vi "Time 1.1-1.2 comparison.vi"() -> ()   [LabVIEW 2013]
panel:
  out "Fib":i32
  out "Time3":dbl
  out "Time2":dbl
  out "f(n)":i32
  out "fib(n)":i32
  out "Time1":dbl
  in  "n":i16
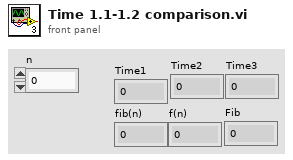
[diagram p1: front panel]
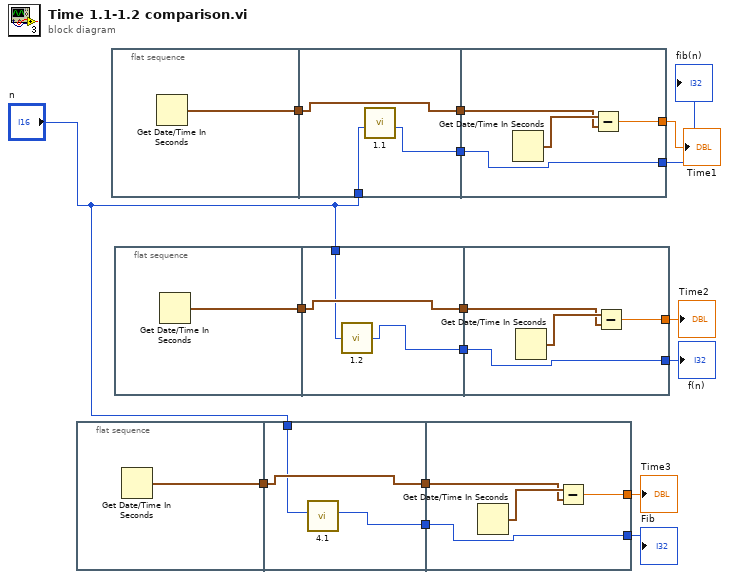
[diagram p0: block diagram]
diagram:
  n1 = flat-sequence {
    tunnel: [w17] -> w6
    tunnel: w6 -> [w20]
    tunnel: [w20] -> w5
    tunnel: [w18] -> w4
    tunnel: "n" -> [w19]
    tunnel: w5 -> [w21]
    tunnel: [w24] -> w3
    tunnel: w4 -> [w23]
    tunnel: [w23] -> w2
    frame #0 {
      n2 = Get Date/Time In Seconds() -> (seconds since 1Jan1904=w17:timestamp)
    }
    frame #1 {
      n3 = call "4.1.vi"("input variable"=w19) -> ("output variable"=w18:i32)  [unwired: 10 in]
    }
    frame #2 {
      n4 = Get Date/Time In Seconds() -> (seconds since 1Jan1904=w22:timestamp)
      n5 = Subtract(x=w22, y=w21) -> (x-y=w24:dbl)
    }
  }
  n6 = flat-sequence {
    tunnel: [w25] -> w16
    tunnel: "n" -> [w28]
    tunnel: w16 -> [w27]
    tunnel: [w27] -> w15
    tunnel: [w26] -> w13
    tunnel: w15 -> [w29]
    tunnel: [w32] -> w14
    tunnel: w13 -> [w31]
    tunnel: [w31] -> w12
    frame #0 {
      n7 = Get Date/Time In Seconds() -> (seconds since 1Jan1904=w25:timestamp)
    }
    frame #1 {
      n8 = call "1.1.vi"("n"=w28) -> ("fib(n)"=w26:i32)  [unwired: 10 in]
    }
    frame #2 {
      n9 = Get Date/Time In Seconds() -> (seconds since 1Jan1904=w30:timestamp)
      n10 = Subtract(x=w30, y=w29) -> (x-y=w32:dbl)
    }
  }
  n11 = flat-sequence {
    tunnel: [w33] -> w11
    tunnel: w11 -> [w36]
    tunnel: [w36] -> w10
    tunnel: [w34] -> w9
    tunnel: "n" -> [w35]
    tunnel: w10 -> [w37]
    tunnel: [w40] -> w7
    tunnel: w9 -> [w39]
    tunnel: [w39] -> w8
    frame #0 {
      n12 = Get Date/Time In Seconds() -> (seconds since 1Jan1904=w33:timestamp)
    }
    frame #1 {
      n13 = call "1.2.vi"("n"=w35) -> ("f(n)"=w34:i32)
    }
    frame #2 {
      n14 = Get Date/Time In Seconds() -> (seconds since 1Jan1904=w38:timestamp)
      n15 = Subtract(x=w38, y=w37) -> (x-y=w40:dbl)
    }
  }
  "Time1" <- w14
  "fib(n)" <- w12
  "f(n)" <- w8
  "Time2" <- w7
  "Time3" <- w3
  "Fib" <- w2
